vi "OutSineReferenceGet.vi"(0 "SR865 in":T2, 5 "error in":errorcluster) -> (14 "SR865 out":T2, 16 "OutSineRef":T1 caption="Out sine ref" items=["Common", "Difference"], 19 "error out":errorcluster)   [LabVIEW 2017]
uses:
  SR865.ctl
  OutSineReference.ctl
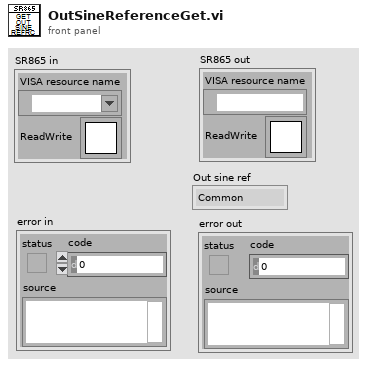
[diagram p1: front panel]
types:
  T1 = typedef "OutSineReference.ctl" = u16
  T2 = typedef "SR865.ctl" = cluster{"VISA resource name":refnum<visa-resource-name>, "ReadWrite":T3}
  T3 = typedef "Semaphore RefNum" = refnum<k1>
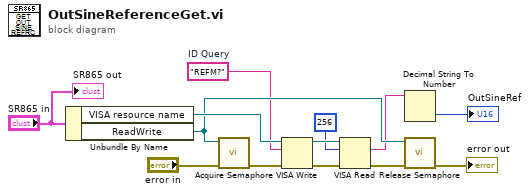
[diagram p0: block diagram]
diagram:
  w2 = "REFM?"  # ID Query
  n1 = Unbundle By Name("SR865 in") -> ("VISA resource name"=w9:refnum<visa-resource-name>, "ReadWrite"=w4:T3)
  n2 = call <vilib>:"Acquire Semaphore.vi"("error in (no error)"="error in", "semaphore"=w4) -> ("error out"=w8:errorcluster)  [unwired: 3 in, 2 out]
  n3 = VISA Write(VISA resource name=w9, write buffer=w2, error in (no error)=w8) -> (VISA resource name out=w12:refnum<visa-resource-name>, error out=w11:errorcluster)  [unwired: 1 out]
  n4 = VISA Read(VISA resource name=w12, byte count=u32 256, error in (no error)=w11) -> (read buffer=w3:string, error out=w6:errorcluster)  [unwired: 2 out]
  n5 = Decimal String To Number(string=w3) -> (number=→"OutSineRef":i32)  [unwired: 2 in, 1 out]
  n6 = call <vilib>:"Release Semaphore.vi"("error in (no error)"=w6, "semaphore"=w4) -> ("error out"=→"error out":errorcluster)  [unwired: 4 in, 1 out]
  "SR865 out" <- "SR865 in"
